vi "started.vi"(8 "error in (no error)":errorcluster, 11 "DIO64Output in":refnum<class "DIO64Output.lvclass">) -> (0 "error out":errorcluster, 2 "started?":bool, 3 "DIO64Output out":refnum<class "DIO64Output.lvclass">)   [LabVIEW 2011, in "Hardware.lvlib" / "Channels.lvlib" / "DIO64Output.lvclass"]
uses:
  DIO64Output.lvclass
  DIO64Output.lvclass/DIO64Output.ctl
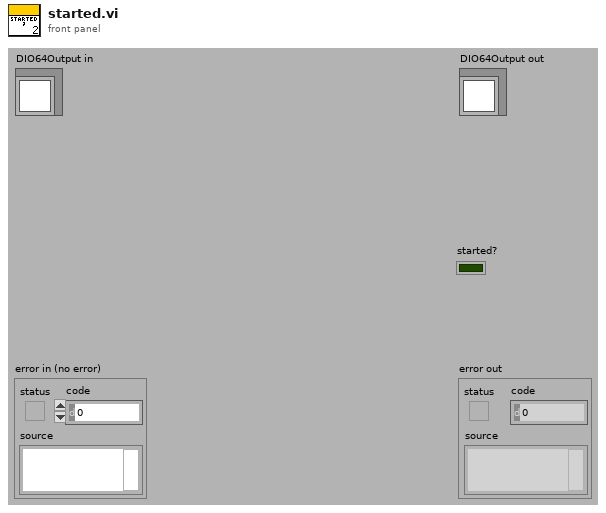
[diagram p1: front panel]
types:
  T1 = typedef "DIO64 Out Status.ctl" = cluster{"pktsize":u16, "portCount":u16, "writePtr":u16, "readPtr":u16, "time0":u16, "time1":u16, "fifoSize":u32, "fifo0":u16, "ticks":u32, "flags":u16, "clkControl":u16, "startControl":u16, "stopControl":u16, "AIControl":u32, "AICurrent":u16, "startTime0":u16, "startTime1":u16, "stopTime0":u16, "stopTime1":u16, "cur trans":u32, "cur reps":u32}
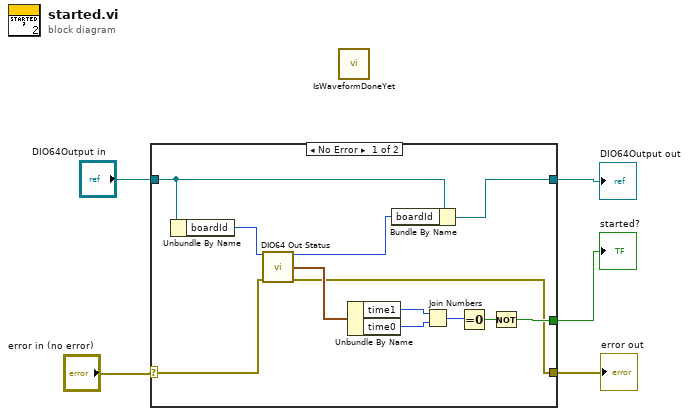
[diagram p0: block diagram]
diagram:
  n1 = case shown="No Error" "error in (no error)" {
    selector: "error in (no error)" -> [w15 w19]
    tunnel: [w9 w19] -> w4
    tunnel: "DIO64Output in" -> [w7 w18]
    tunnel: [w6 w18] -> w2
    tunnel: [w10 _] -> w1
    frame No Error {
      n2 = Unbundle By Name(w7) -> ("boardId"=w16:i32)
      n3 = call <userlib>:"DIO64 Out Status.vi"("board in"=w16, "error in (no error)"=w15) -> ("board out"=w8:u16, "Out Status"=w17:T1, "error out"=w9:errorcluster)  [unwired: 10 in, 1 out]
      n4 = Unbundle By Name(w17) -> ("time1"=w14:u16, "time0"=w13:u16)
      n5 = Bundle By Name(cluster=w7, "boardId"=w8) -> (w6:refnum<class "DIO64Output.lvclass">)
      n6 = Join Numbers(hi=w14, lo=w13) -> ((hi.lo)=w12:u32)
      n7 = Equal To 0?(x=w12) -> (x = 0?=w11:bool)
      n8 = Not(x=w11) -> (.not. x?=w10:bool)
    }
    frame Error {
    }
  }
  "error out" <- w4
  "DIO64Output out" <- w2
  "started?" <- w1
  n9 = call <userlib>:"IsWaveformDoneYet.vi"() -> ()  [unwired: 13 in, 3 out]
